vi "Module Cleanup.vi"(8 "error in (no error)":errorcluster, 11 "SlowCalcs Module in":refnum<class "SlowCalcs Module.lvclass">) -> (0 "error out":errorcluster, 3 "SlowCalcs Module out":refnum<class "SlowCalcs Module.lvclass">)   [LabVIEW 2020, in "VolatusCalcs.lvlib" / "SlowCalcs Module.lvclass"]
uses:
  SlowCalcs Module.lvclass
  SlowCalcs Module.lvclass/SlowCalcs Module.ctl
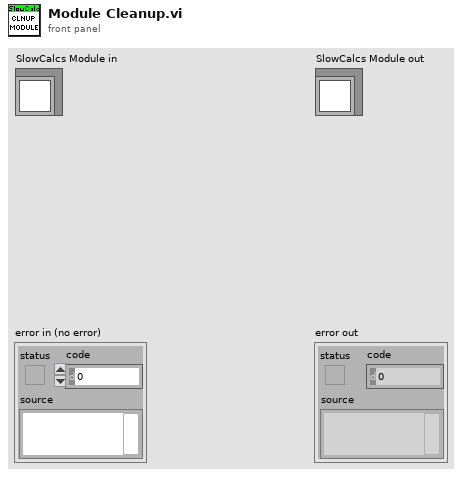
[diagram p1: front panel]
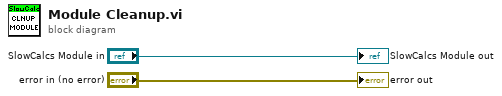
[diagram p0: block diagram]
diagram:
  "error out" <- "error in (no error)"
  "SlowCalcs Module out" <- "SlowCalcs Module in"
